vi "R1DOControl_Manual.vi"(7 "LabVIEW Web Service Request":refnum<class "Web Request.lvclass">, 9 "N2MFC":dbl, 11 "AirMFC":dbl) -> (2 "ControlStatus":string, 3 "R1_DO_Manual":cluster{"Air MFC":dbl, "N2 MFC":dbl})   [LabVIEW 2016]
uses:
  <vilib>/wsapi/Web Request.lvclass
panel:
  # "Use the Web Service Request input terminal to call the VIs on the Web Services palette. Do not remove it from the connector pane unless you don't need access to the palette."
  # "Each additional control wired to the connector pane will be available as an input in the URL. To include an indicator in terminal-mode output (the default setting), it must also be wired to the connector pane."
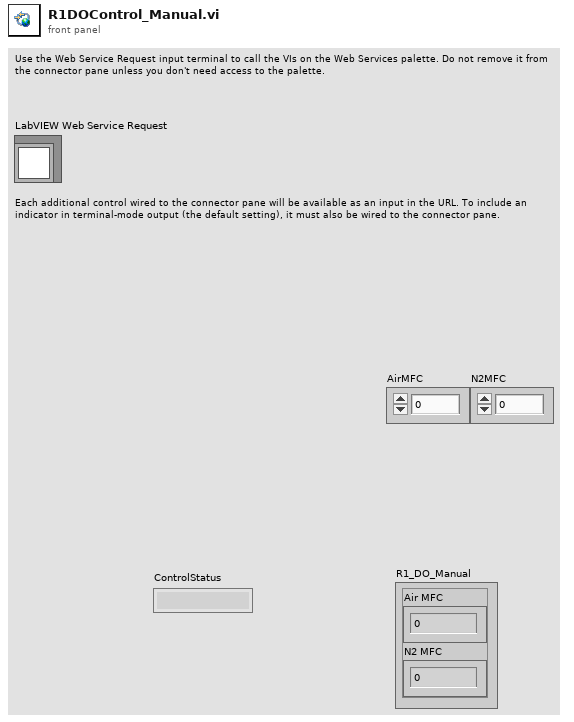
[diagram p1: front panel]
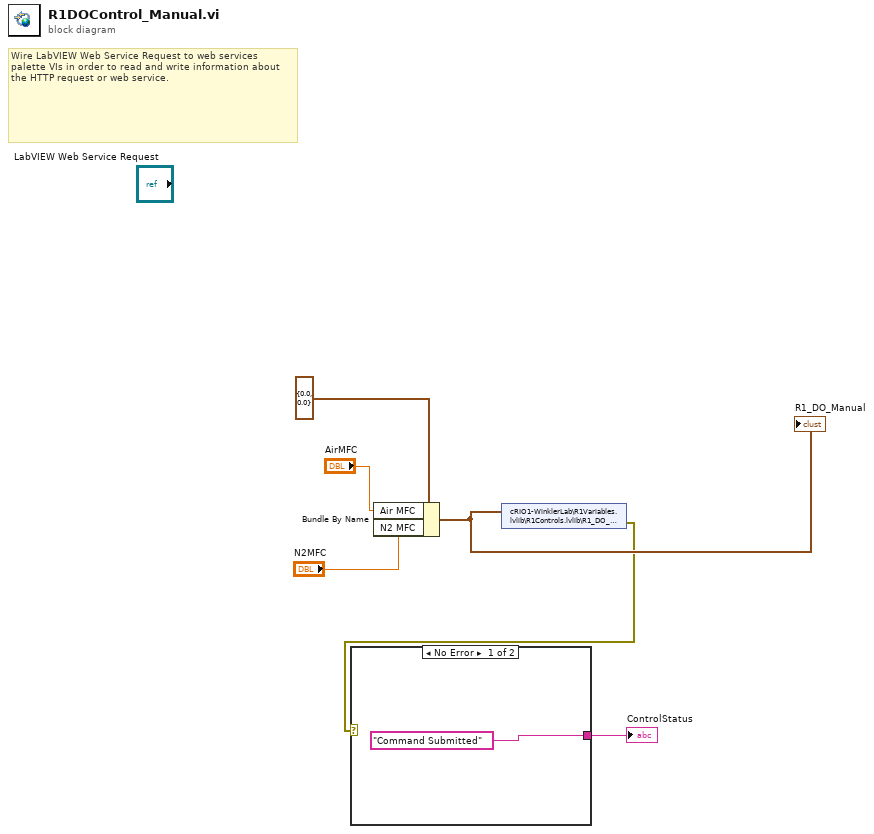
[diagram p0: block diagram]
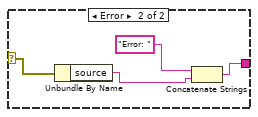
[diagram p2: hidden frame]
diagram:
  # "Wire LabVIEW Web Service Request to web services palette VIs in order to read and write information about the HTTP request or web service."
  n1 = Bundle By Name(cluster=cluster{"Air MFC":dbl, "N2 MFC":dbl} {"Air MFC"=0.0, "N2 MFC"=0.0} ("R1_DO_Manual"), "Air MFC"="AirMFC", "N2 MFC"="N2MFC") -> (w6:cluster{"Air MFC":dbl, "N2 MFC":dbl})
  "R1_DO_Manual" <- w6
  n2 = shared-variable "cRIO1-WinklerLab\\R1Variables.lvlib\\R1Controls.lvlib\\R1_DO_Manual"(w6) -> (error out=w2:errorcluster)  [unwired: 1 in]
  n3 = case shown="No Error" w2 {
    selector: w2 -> [_ w9]
    tunnel: ["Command Submitted" ("ControlStatus") w8] -> w1
    frame No Error {
    }
    frame Error {
      n4 = Unbundle By Name(w9) -> ("source"=w11:string)
      n5 = Concatenate Strings("Error: ", w11) -> (w8:string)
    }
  }
  "ControlStatus" <- w1
